vi "ReadConfigClusterComplex.vi"(0 "Configfile input":T1, 1 "Cluster 2":refnum<vi>, 2 "error in (no error)":errorcluster) -> (3 "refnum out":T1, 4 "reference out":refnum<vi>, 5 "err":bool, 6 "error out":errorcluster)   [LabVIEW 2009]
uses:
  <vilib>/Utility/config.llb/Config Data RefNum.ctl
  Read Key (String).vi
  <vilib>/Utility/config.llb/NI_LVConfig.lvlib
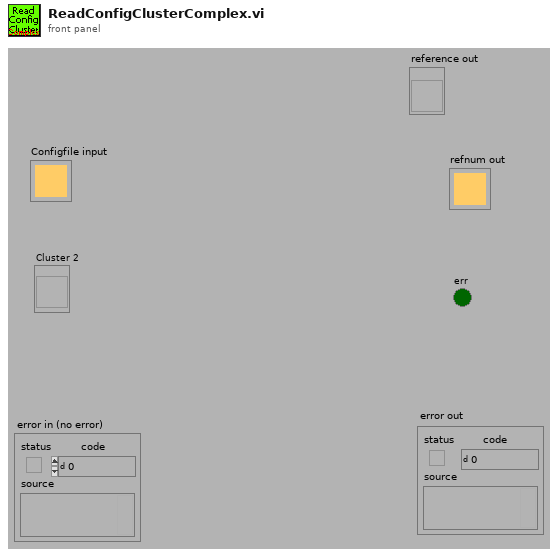
[diagram p1: front panel]
types:
  T1 = typedef "NI_LVConfig.lvlib/Config Data RefNum.ctl" = refnum<k1>
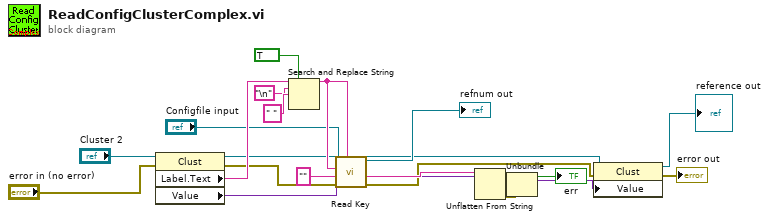
[diagram p0: block diagram]
diagram:
  n1 = property class="Clust"(reference="Cluster 2", error in="error in (no error)") -> (reference out=w7:refnum<vi>, error out=w10:errorcluster, "Label.Text"=w16:string, "Value"=w11:variant)
  n2 = Search and Replace String(replace all?=TRUE ("replace all? (F)"), input string=w16, search string="\n", replace string=" " ("replace string (\"\")")) -> (result string=w15:string)  [unwired: 4 in, 3 out]
  n3 = call-poly "Read Key.vi"("section"=w15, "error in (no error)"=w10, "default value"="", "key"=w15, "refnum"="Configfile input") -> ("error out"=w3:errorcluster, "value"=w13:string, "refnum out"=→"refnum out":T1)  [unwired: 3 in, 1 out]
  n4 = Unflatten From String(type=w11, binary string=w13) -> (value=w6:variant, error out=w2:errorcluster)  [unwired: 3 in, 1 out]
  n5 = Unbundle(w2) -> ("status"=→"err":bool)  [unwired: 2 out]
  n6 = property class="Clust"(reference=w7, error in=w3, "Value"=w6) -> (reference out=→"reference out":refnum<vi>, error out=→"error out":errorcluster)
